vi "User_generated_event.vi"() -> ()   [LabVIEW 2020]
panel:
  out "error out":errorcluster
  in  "Switch":bool
  in  "error in (no error)":errorcluster
  out "Action":string
  in  "Stop":bool
  in  "Input Text":string
  in  "Input Num":dbl
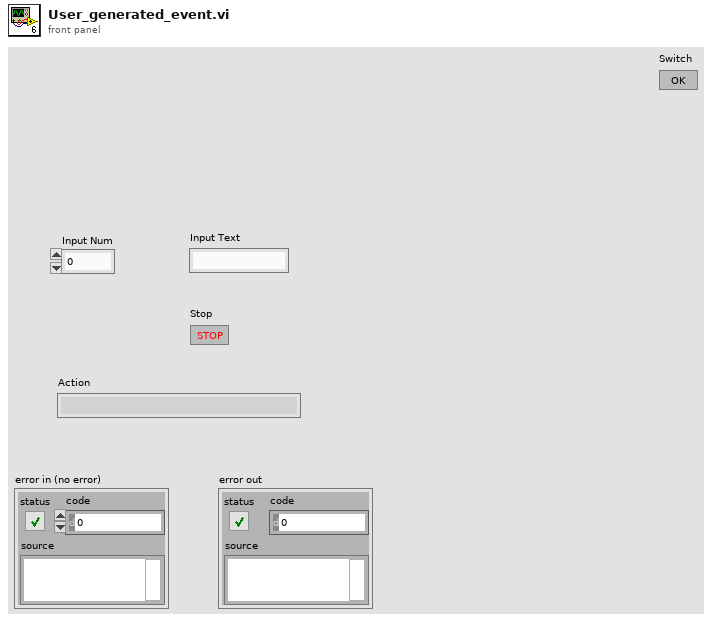
[diagram p1: front panel]
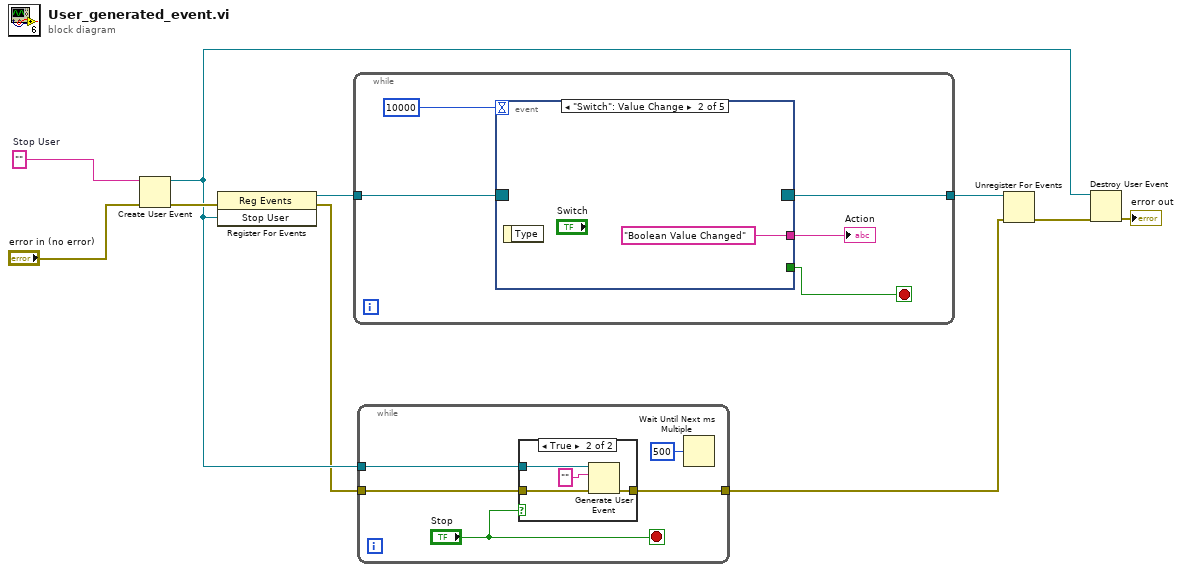
[diagram p0: block diagram]
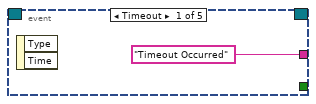
[diagram p3: hidden frame]
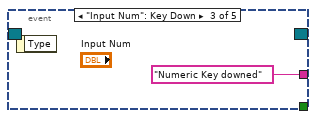
[diagram p4: hidden frame]
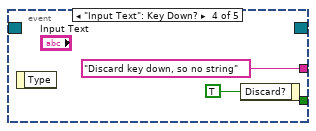
[diagram p5: hidden frame]
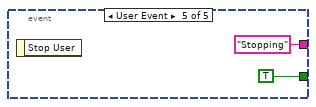
[diagram p6: hidden frame]
diagram:
  w3 = ""  # Stop User
  n1 = Create User Event(user event datatype=w3, error in="error in (no error)") -> (user event=w7:refnum<user-event>, error out=w9:errorcluster)
  n2 = register-events(error in=w9, w7) -> (reference out=w8:refnum<event-registration>, error out=w6:errorcluster)  [unwired: 1 in]
  n3 = while {
    tunnel: w8 -> [w12]
    tunnel: [w11] -> w1
    stop <- w13 stop-if-true
    n4 = event shown="[1] \"Switch\": Value Change" {
      selector: w12 -> [_ _ _ _ _]
      dyn-events: [_ _ _ _ _] -> w11
      timeout: 10000 -> [_ _ _ _ _]
      tunnel: ["Timeout Occurred" "Boolean Value Changed" "Numeric Key downed" "Discard key down, so no string" "Stopping"] -> w14
      tunnel: [_ _ _ _ TRUE] -> w13
      event Timeout {
        n5 = event-data() -> ()  [unwired: 1 in, 2 out]
      }
      event "Switch": Value Change {
        n6 = event-data() -> ()  [unwired: 1 in, 1 out]
      }
      event "Input Num": Key Down {
        n7 = event-data() -> ()  [unwired: 1 in, 1 out]
      }
      event "Input Text": Key Down? {
        n8 = event-data() -> ()  [unwired: 1 in, 1 out]
        n9 = event-data("Discard?"=TRUE) -> ()  [unwired: 1 in, 1 out]
      }
      event User Event {
        n10 = event-data() -> ()  [unwired: 1 in, 1 out]
      }
    }
    "Action" <- w14
  }
  n11 = while {
    tunnel: w7 -> [w27]
    tunnel: w6 -> [w26]
    tunnel: [w23] -> w5
    stop <- "Stop" stop-if-true
    n12 = case shown="True" "Stop" {
      tunnel: w27 -> [_ w32]
      tunnel: w26 -> [w28 w31]
      tunnel: [w28 w29] -> w23
      frame False {
      }
      frame True {
        n13 = Generate User Event(user event=w32, event data cluster="" ("event data"), error in=w31) -> (error out=w29:errorcluster)  [unwired: 1 in, 1 out]
      }
    }
    n14 = Wait Until Next ms Multiple(millisecond multiple=u32 500) -> ()  [unwired: 1 out]
  }
  n15 = Unregister For Events(event registration refnum=w1, error in=w5) -> (error out=w4:errorcluster)
  n16 = Destroy User Event(user event=w7, error in=w4) -> (error out=→"error out":errorcluster)
